vi "Basic Interface.vi"() -> ()   [LabVIEW 2019]
uses:
  source code/LSL components/scripts/scripts manager/scripts manager.lvclass
  source code/LSL components/output terminal/Plain OT/PainOutputTerminal.lvclass
  C:/Users/Patrick/Documents/GitHub/LabVIEW-Script-Language/source code/LSL components/output terminal/Base/Output Terminal.lvclass
  source code/LSL components/output terminal/Plain OT/PainOutputTerminal.lvclass/PainOutputTerminal.ctl
  source code/LSL components/variables/RT Variables/RT Variables.lvclass
  source code/LSL components/scripts/scripts manager/scripts manager.lvclass/scripts manager.ctl
  a3015e6c-1936-464d-a698-599e3c554b07.vi
  source code/LSL components/output terminal/Plain OT/properties/Write Output Terminal.vi
  source code/LSL components/scripts/scripts manager/properties/Write Scripts.vi
panel:
  in  "Script Editor":string
  in  "Path":path
  in  "Help":bool
  in  "Script Compile":bool
  in  "Script Save":bool
  in  "Script Delete":bool
  in  "Script New":bool
  in  "Script Run":bool
  in  "Script Files":i32(listbox)
  out "Output Terminal":string
  in  "Script Line":string
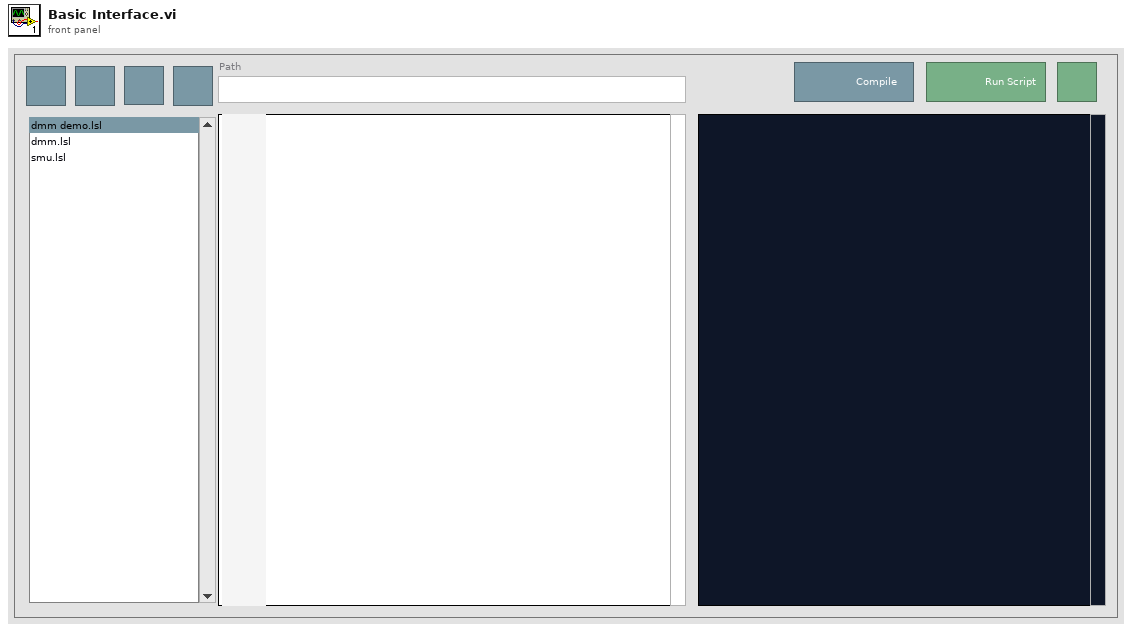
[diagram p1: front panel]
types:
  T1 = enum32{"Invalid", "Standard", "Closed", "Hidden", "Minimized", "Maximized"}
  T2 = enum32{"invalid app kind", "Development System", "Run Time System", "Student Edition", "Embedded LabVIEW", "Evaluation", "Custom"}
  T3 = cluster{"Core":cluster{"Current VI Reference":refnum<vi>, "Close Panel on Exit?":bool}, "scripts manager":refnum<class "scripts manager.lvclass">, "Script":string, "Script Folder":path, "Script Filename":string, "PainOT":refnum<class "PainOutputTerminal.lvclass">}
  T4 = cluster{"Current VI Reference":refnum<vi>, "Close Panel on Exit?":bool}
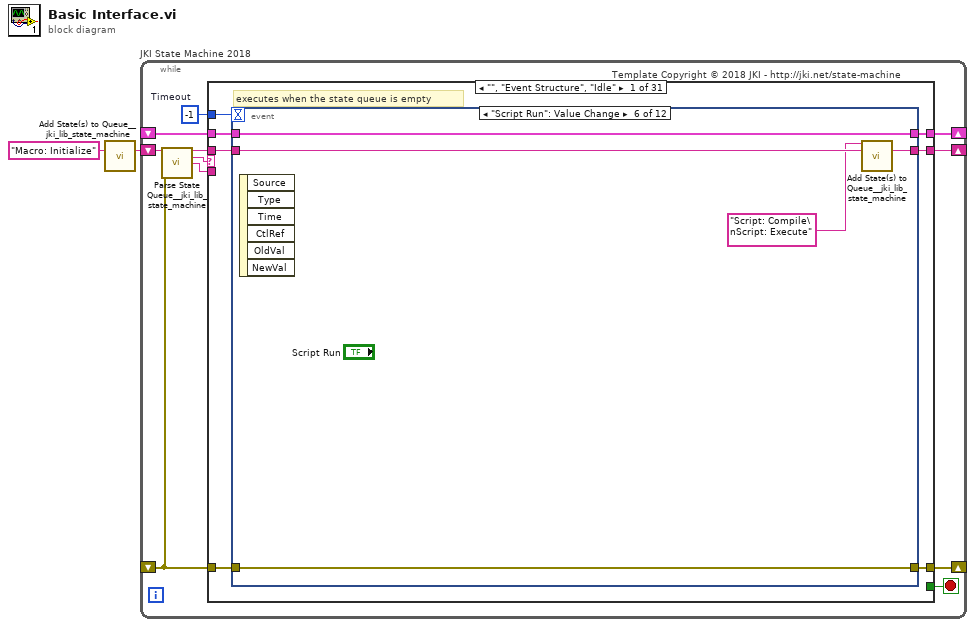
[diagram p0: block diagram]
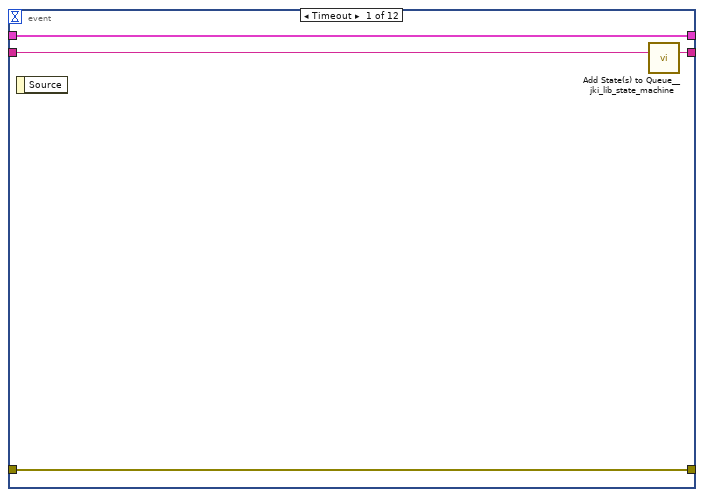
[diagram p2: hidden frame]
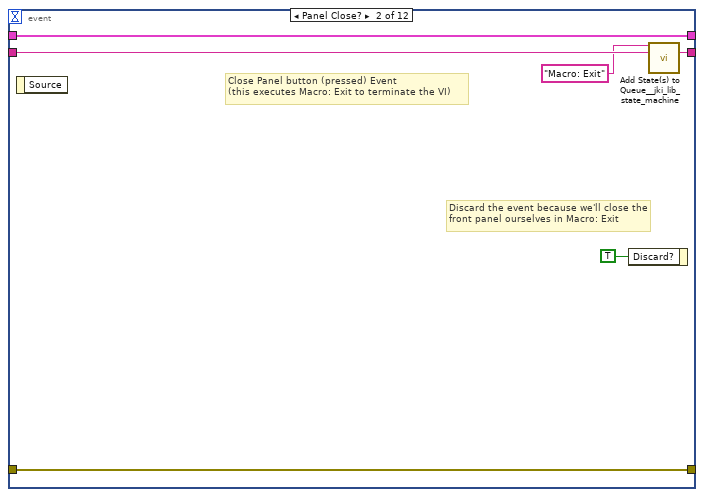
[diagram p3: hidden frame]
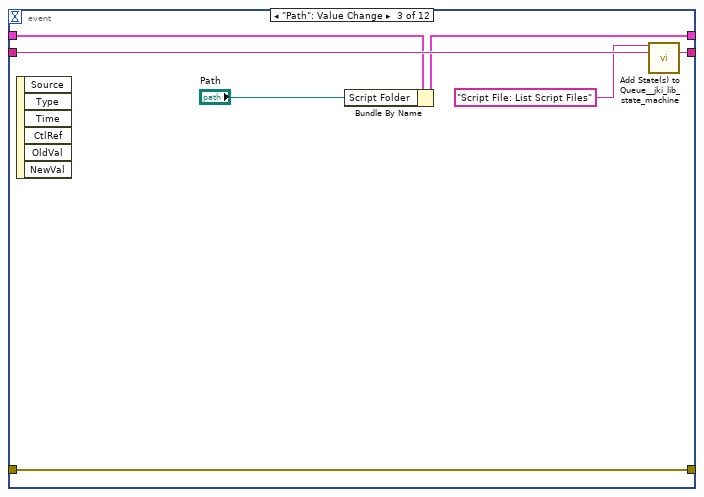
[diagram p4: hidden frame]
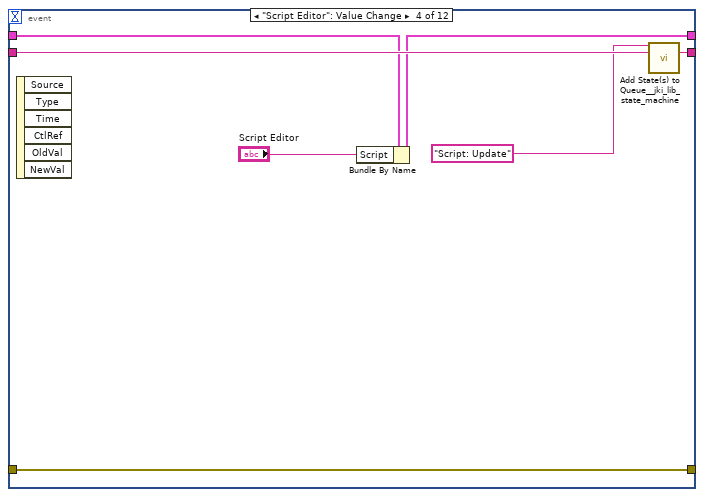
[diagram p5: hidden frame]
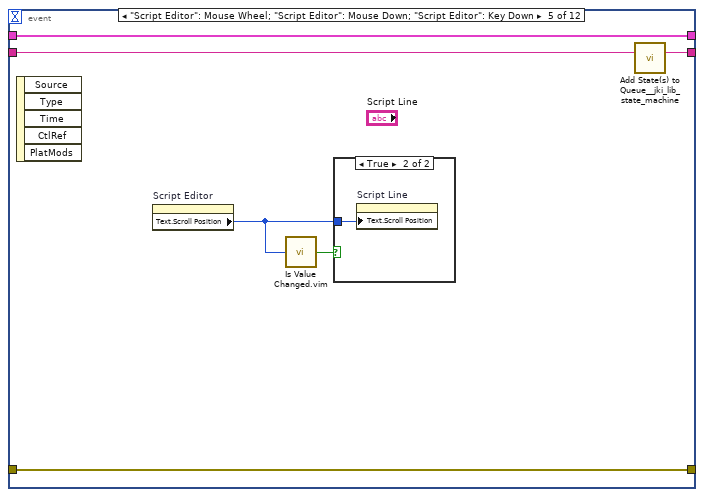
[diagram p6: hidden frame]
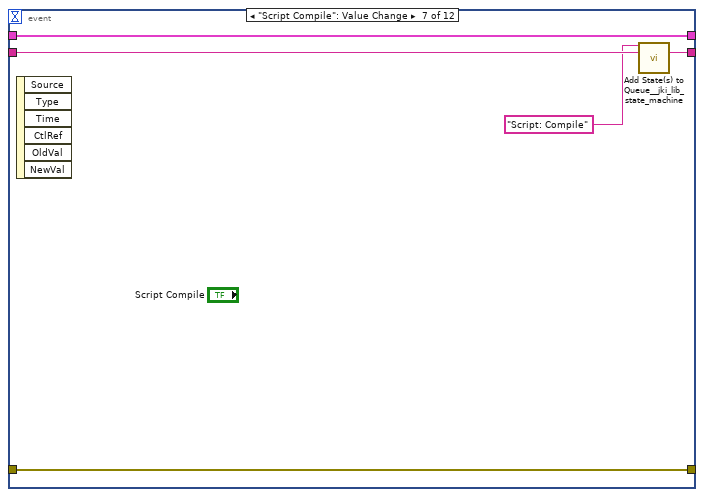
[diagram p8: hidden frame]
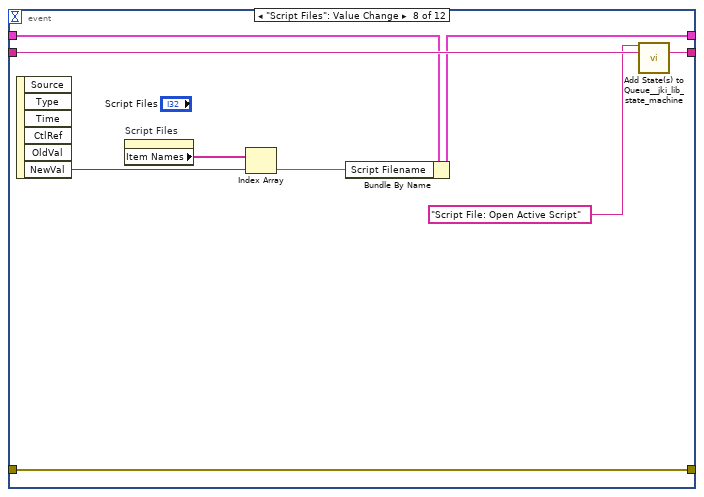
[diagram p9: hidden frame]
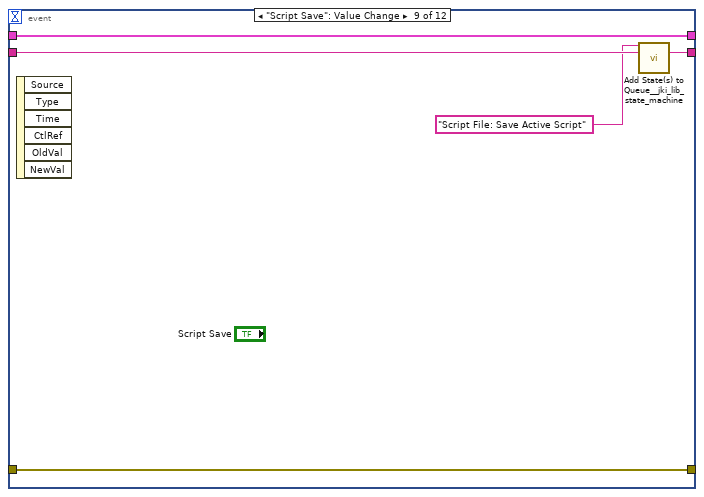
[diagram p10: hidden frame]
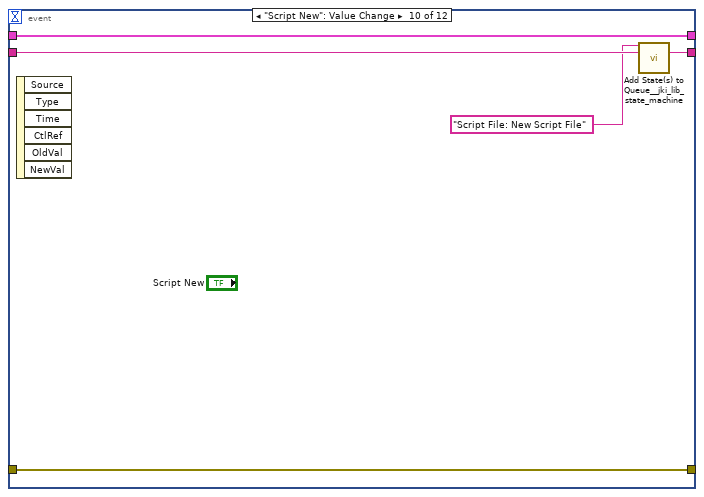
[diagram p11: hidden frame]
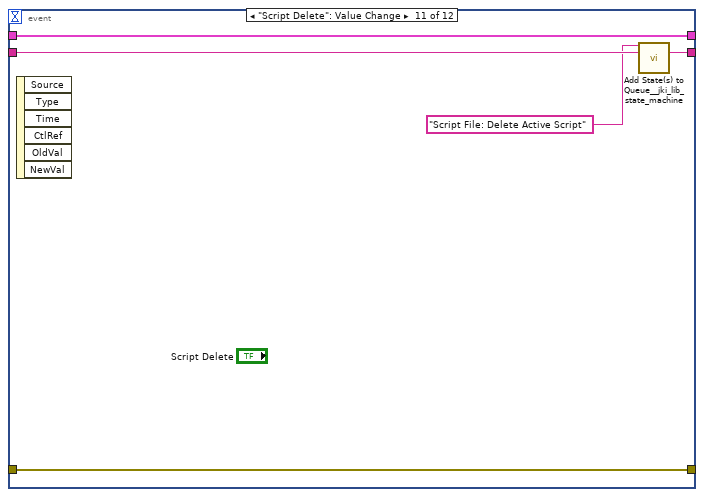
[diagram p12: hidden frame]
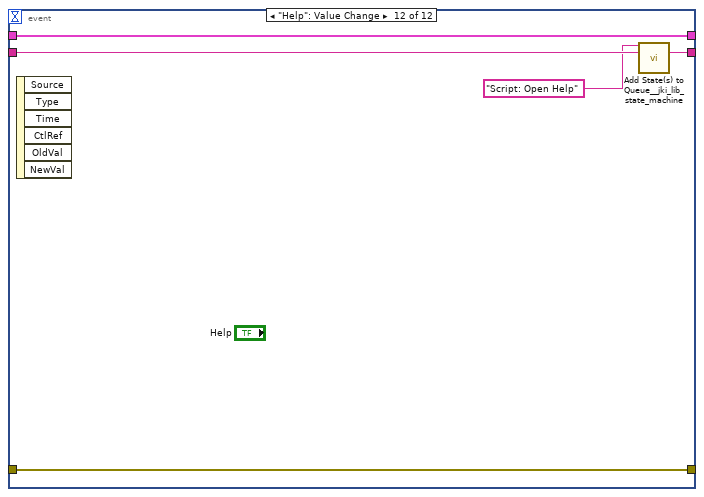
[diagram p13: hidden frame]
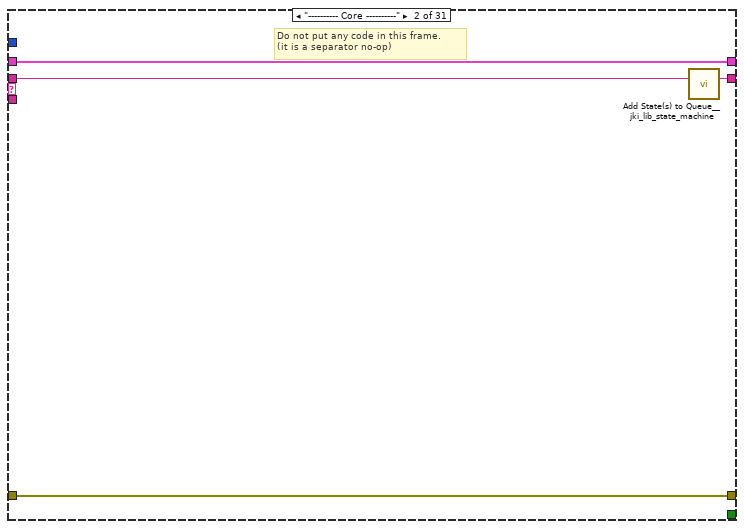
[diagram p14: hidden frame]
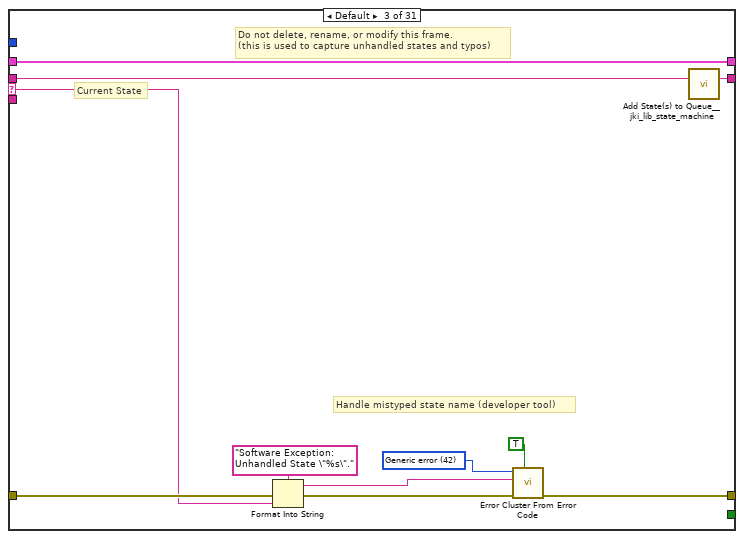
[diagram p15: hidden frame]
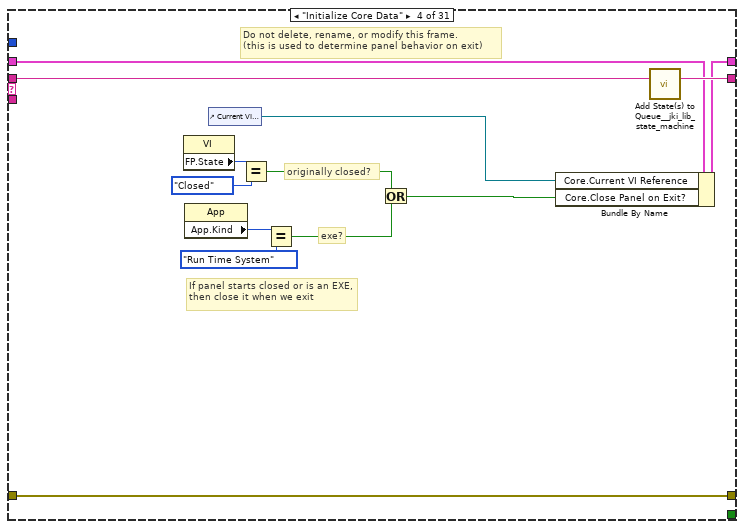
[diagram p16: hidden frame]
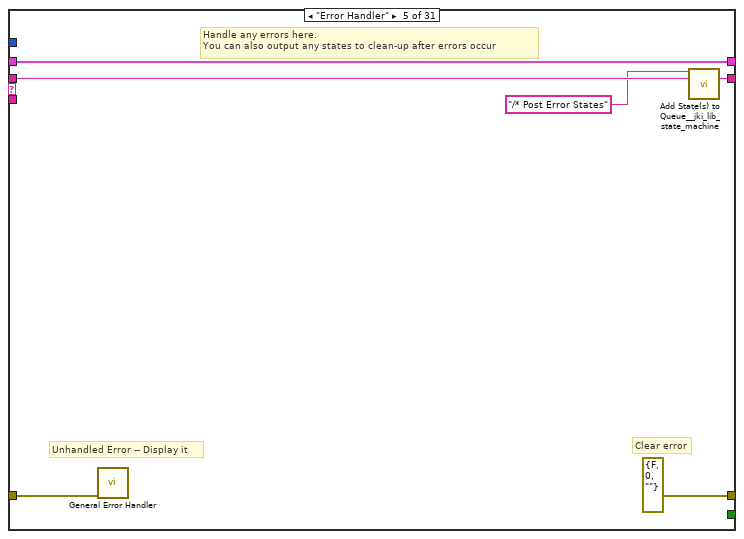
[diagram p17: hidden frame]
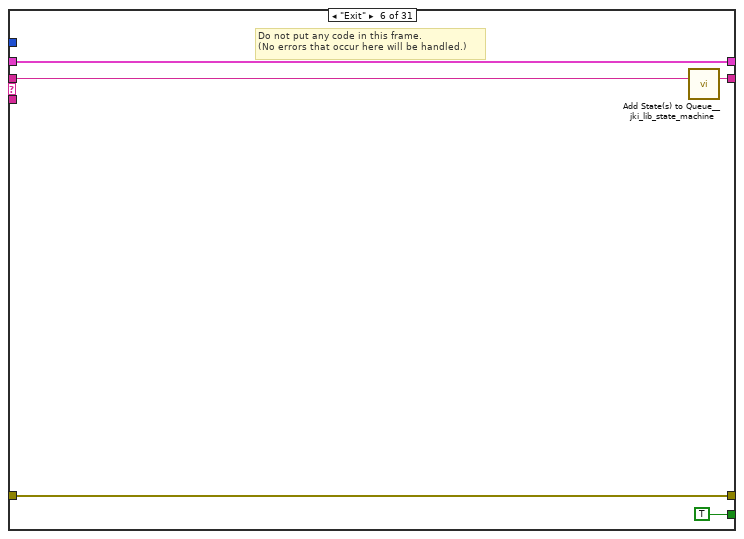
[diagram p18: hidden frame]
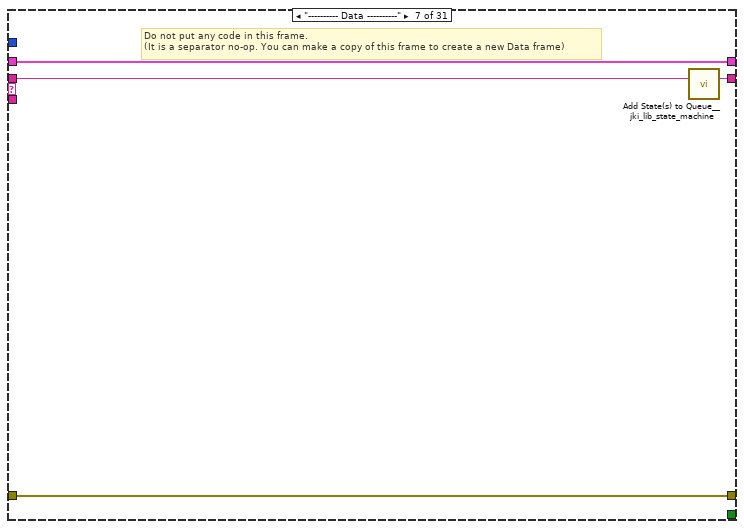
[diagram p19: hidden frame]
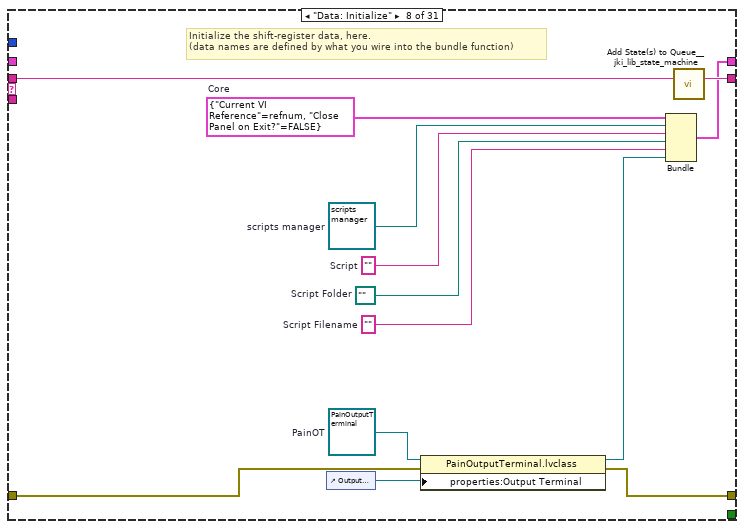
[diagram p20: hidden frame]
diagram:
  n1 = call <vilib>:"Add State(s) to Queue__jki_lib_state_machine.vi"("State(s) in (\"\")"="Macro: Initialize") -> ("States Out"=w2:string)  [unwired: 14 in]
  n2 = while "JKI State Machine 2018" {
    shift-right: [w6] -> _
    shift-left: _ -> [w5]
    shift-right: [w9] -> _
    shift-left: _ -> [w3]
    shift-right: [w8] -> _
    shift-left: w2 -> [w10]
    stop <- w7 stop-if-true
    w4 = -1  # Timeout
    # "Template Copyright © 2018 JKI - http://jki.net/state-machine"
    n3 = call <vilib>:"Parse State Queue__jki_lib_state_machine.vi"("State Queue"=w10, "Error In (no error)"=w3) -> ("Remaining States"=w12:string, "Current State"=w13:string, "Arguments"=w11:string)  [unwired: 11 in]
    n4 = case shown="\"\", \"Event Structure\", \"Idle\"" w13 {
      selector: w13 -> [_ _ w95 _ _ _ _ _ _ _ _ _ _ _ _ _ _ _ _ _ _ _ _ _ _ _ _ _ _ _ _]
      tunnel: w12 -> [w20 w94 w99 w118 w124 w129 w133 w146 w162 w187 w191 w203 w209 w220 w289 w294 w304 w310 w320 w329 w337 w345 w353 w358 w362 w373 w446 w456 w466 w478 w499]
      tunnel: w11 -> [_ _ _ _ _ _ _ _ _ _ _ _ w204 w214 _ _ _ _ _ _ _ _ _ _ _ w367 _ _ _ _ _]
      tunnel: w5 -> [w18 w91 w97 w111 w121 w127 w130 _ w151 w182 w188 w201 w207 w216 w286 w291 w301 w306 w317 w326 w334 w342 w350 w356 w359 w366 w444 w454 w464 w476 w497]
      tunnel: [w17 w92 w101 w115 errorcluster {"status"=FALSE, "code"=0, "source"=""} ("error out") w126 w131 w139 w150 w183 w189 w194 w205 w217 w287 w292 w302 w308 w314 w322 w332 w341 w347 w355 w360 w364 w438 w449 w462 w471 w491] -> w9
      tunnel: w3 -> [w16 w92 w100 w115 w120 w126 w131 w138 w149 w184 w189 w193 w206 w218 w287 w292 w302 w308 w313 w321 w331 w339 w346 w354 w360 w363 w437 w448 w457 w470 w490]
      tunnel: [w19 w93 w98 w117 w123 w128 w132 w145 w161 w186 w190 w202 w208 w219 w288 w293 w303 w309 w319 w328 w336 w344 w352 w357 w361 w372 w445 w455 w465 w477 w498] -> w8
      tunnel: [_ _ _ _ _ TRUE _ _ _ _ _ _ _ _ _ _ _ _ _ _ _ _ _ _ _ _ _ _ _ _ _] -> w7
      tunnel: [w15 w91 w97 w116 w121 w127 w130 w144 w152 w182 w188 w201 w207 w216 w286 w291 w301 w307 w318 w327 w335 w343 w351 w356 w359 w366 w444 w454 w464 w476 w497] -> w6
      tunnel: w4 -> [w14 _ _ _ _ _ _ _ _ _ _ _ _ _ _ _ _ _ _ _ _ _ _ _ _ _ _ _ _ _ _]
      frame "", "Event Structure", "Idle" {
        # "executes when the state queue is empty"
        n5 = event shown="[5] \"Script Run\": Value Change" {
          selector: _ -> [_ _ _ _ _ _ _ _ _ _ _ _]
          dyn-events: _ -> [_ _ _ _ _ _ _ _ _ _ _ _]
          timeout: w14 -> [_ _ _ _ _ _ _ _ _ _ _ _]
          tunnel: w20 -> [w24 w30 w37 w44 w49 w54 w59 w69 w73 w78 w83 w88]
          tunnel: [w23 w29 w36 w43 w50 w55 w60 w70 w74 w79 w84 w89] -> w19
          tunnel: w18 -> [w21 w27 w32 w39 w48 w56 w61 w65 w75 w80 w85 w90]
          tunnel: [w22 w28 w35 w42 w47 w52 w57 w67 w71 w76 w81 w86] -> w17
          tunnel: w16 -> [w22 w28 w35 w42 w47 w52 w57 w67 w71 w76 w81 w86]
          tunnel: [w21 w27 w33 w40 w48 w56 w61 w66 w75 w80 w85 w90] -> w15
          event Timeout {
            n6 = event-data() -> ()  [unwired: 1 in, 1 out]
            n7 = call <vilib>:"Add State(s) to Queue__jki_lib_state_machine.vi"("State(s) in (\"\")"=w24) -> ("States Out"=w23:string)  [unwired: 14 in]
          }
          event Panel Close? {
            # "Discard the event because we'll close the front panel ourselves in Macro: Exit"
            # "Close Panel button (pressed) Event\n(this executes Macro: Exit to terminate the VI)"
            n8 = event-data() -> ()  [unwired: 1 in, 1 out]
            n9 = event-data("Discard?"=TRUE) -> ()  [unwired: 1 in, 1 out]
            n10 = call <vilib>:"Add State(s) to Queue__jki_lib_state_machine.vi"("State(s) in Front (\"\")"="Macro: Exit", "State(s) in (\"\")"=w30) -> ("States Out"=w29:string)  [unwired: 13 in]
          }
          event "Path": Value Change {
            n11 = event-data() -> ()  [unwired: 1 in, 6 out]
            n12 = Bundle By Name(cluster=w32, "Script Folder"="Path") -> (w33:T3)
            n13 = call <vilib>:"Add State(s) to Queue__jki_lib_state_machine.vi"("State(s) in Front (\"\")"="Script File: List Script Files", "State(s) in (\"\")"=w37) -> ("States Out"=w36:string)  [unwired: 13 in]
          }
          event "Script Editor": Value Change {
            n14 = event-data() -> ()  [unwired: 1 in, 6 out]
            n15 = Bundle By Name(cluster=w39, "Script"="Script Editor") -> (w40:T3)
            n16 = call <vilib>:"Add State(s) to Queue__jki_lib_state_machine.vi"("State(s) in Front (\"\")"="Script: Update", "State(s) in (\"\")"=w44) -> ("States Out"=w43:string)  [unwired: 13 in]
          }
          event "Script Editor": Mouse Wheel; "Script Editor": Mouse Down; "Script Editor": Key Down {
            n17 = event-data() -> ()  [unwired: 1 in, 5 out]
            n18 = property on="Script Editor" class="Str"() -> ("Text.Scroll Position"=w46:u32)  [unwired: 2 in, 2 out]
            n19 = call "Is Value Changed.vim"("value"=w46) -> ("changed or first call?"=w45:bool)
            n20 = case shown="True" w45 {
              tunnel: w46 -> [_ w51]
              frame False {
              }
              frame True {
                n21 = property on="Script Line" class="Str"("Text.Scroll Position"=w51) -> ()  [unwired: 2 in, 2 out]
              }
            }
            n22 = call <vilib>:"Add State(s) to Queue__jki_lib_state_machine.vi"("State(s) in (\"\")"=w49) -> ("States Out"=w50:string)  [unwired: 14 in]
          }
          event "Script Run": Value Change {
            n23 = event-data() -> ()  [unwired: 1 in, 6 out]
            n24 = call <vilib>:"Add State(s) to Queue__jki_lib_state_machine.vi"("State(s) in Front (\"\")"="Script: Compile\nScript: Execute" ("State(s) at Back (\"\")"), "State(s) in (\"\")"=w54) -> ("States Out"=w55:string)  [unwired: 13 in]
          }
          event "Script Compile": Value Change {
            n25 = event-data() -> ()  [unwired: 1 in, 6 out]
            n26 = call <vilib>:"Add State(s) to Queue__jki_lib_state_machine.vi"("State(s) in Front (\"\")"="Script: Compile" ("State(s) at Back (\"\")"), "State(s) in (\"\")"=w59) -> ("States Out"=w60:string)  [unwired: 13 in]
          }
          event "Script Files": Value Change {
            n27 = event-data() -> ("NewVal"=w62:i32)  [unwired: 1 in, 5 out]
            n28 = property on="Script Files" class="LstBox (strict)"() -> ("Item Names"=w64:string[])  [unwired: 2 in, 2 out]
            n29 = Index Array(array=w64, index=w62) -> (element=w63:string)
            n30 = Bundle By Name(cluster=w65, "Script Filename"=w63) -> (w66:T3)
            n31 = call <vilib>:"Add State(s) to Queue__jki_lib_state_machine.vi"("State(s) in Front (\"\")"="Script File: Open Active Script" ("State(s) at Back (\"\")"), "State(s) in (\"\")"=w69) -> ("States Out"=w70:string)  [unwired: 13 in]
          }
          event "Script Save": Value Change {
            n32 = event-data() -> ()  [unwired: 1 in, 6 out]
            n33 = call <vilib>:"Add State(s) to Queue__jki_lib_state_machine.vi"("State(s) in Front (\"\")"="Script File: Save Active Script" ("State(s) at Back (\"\")"), "State(s) in (\"\")"=w73) -> ("States Out"=w74:string)  [unwired: 13 in]
          }
          event "Script New": Value Change {
            n34 = event-data() -> ()  [unwired: 1 in, 6 out]
            n35 = call <vilib>:"Add State(s) to Queue__jki_lib_state_machine.vi"("State(s) in Front (\"\")"="Script File: New Script File" ("State(s) at Back (\"\")"), "State(s) in (\"\")"=w78) -> ("States Out"=w79:string)  [unwired: 13 in]
          }
          event "Script Delete": Value Change {
            n36 = event-data() -> ()  [unwired: 1 in, 6 out]
            n37 = call <vilib>:"Add State(s) to Queue__jki_lib_state_machine.vi"("State(s) in Front (\"\")"="Script File: Delete Active Script" ("State(s) at Back (\"\")"), "State(s) in (\"\")"=w83) -> ("States Out"=w84:string)  [unwired: 13 in]
          }
          event "Help": Value Change {
            n38 = event-data() -> ()  [unwired: 1 in, 6 out]
            n39 = call <vilib>:"Add State(s) to Queue__jki_lib_state_machine.vi"("State(s) in Front (\"\")"="Script: Open Help" ("State(s) at Back (\"\")"), "State(s) in (\"\")"=w88) -> ("States Out"=w89:string)  [unwired: 13 in]
          }
        }
      }
      frame "---------- Core ----------" {
        # "Do not put any code in this frame.\n(it is a separator no-op)"
        n40 = call <vilib>:"Add State(s) to Queue__jki_lib_state_machine.vi"("State(s) in (\"\")"=w94) -> ("States Out"=w93:string)  [unwired: 14 in]
      }
      frame Default {
        w104 = 42 items=["No error", "Argument error", "Memory is full", "Out of zone", "End of file", "File already open", "Generic file I/O error", "File not found", "File permission error", "Disk is full", "Duplicate path", "Too many files open", "System feature not enabled", "Resource file not found", "Cannot add resource", "Resource not found", "Image not found", "Image memory error", "Pen does not exist", "Config type invalid", "Config token not found", "Config parse error", "Config memory error", "Bad external code format", "Bad external code offset", "External code not present", "Null window", "Destroy window error", "Null menu", "Print aborted", "Bad print record", "Print driver error", "Windows error during printing", "Memory error during printing", "Print dialog error", "Generic print error", "Invalid device refnum", "Device not found", "Device parameter error", "Device unit error", "Cannot open device", "Device call aborted", "Generic error", "Cancelled by user", "Object ID too low", "Object ID too high", "Object not in heap", "Unknown heap", "Unknown object (invalid DefProc)", "Unknown object (DefProc not in table)", "Message out of range", "Invalid (null) method", "Unknown message", "Manager call not supported", "Bad address", "Network operation in progress", "Network operation timed out", "Connection is busy", "Network attribute not supported", "Network error", "Address in use", "System out of memory", "Connection aborted", "Connection refused", "Not connected", "Already connected", "Connection closed", "Initialization error (interapplication manager)", "Bad occurrence", "Wait on unbound occurrence handler", "Occurrence queue overflow", "Datalog type conflict", "Unused", "Unrecognized type (interapplication manager)", "Memory corrupt", "Failed to make temporary DLL", "Old CIN version", "Drag socket not found", "Failed to load drop-object", "Failed to register OLE object", "Failed to release OLE object", "Format specifier type mismatch", "Unknown format specifier", "Too few format specifiers", "Too many format specifiers", "Scan failed", "Newer CIN version", "Error converting to variant", "Runtime menu error", "Password tampered", "Variant attribute not found", "Incompatible variant data type", "Event data is not available", "Event Store is not present", "Occurrence is not found", "Event Queue is not created", "Event info is not available", "Refnum passed is NULL", "Error retrieving Class GUID", "Error retrieving CoClass GUID", "Error retrieving TypeLib GUID.", "Bad built application magic bytes.", "Specific driver is different from the specific driver associated with the Logical Name.", "There is no session opened to the class driver.", "Max Error", "MAX - Error with config objects", "MAX - Error loading configuration", "MAX - Group not supported"]
        # "Current State"
        # "Do not delete, rename, or modify this frame.\n(this is used to capture unhandled states and typos)"
        # "Handle mistyped state name (developer tool)"
        n41 = Format Into String(format string="Software Exception: Unhandled State \"%s\"." ("message"), error in=w100, w95) -> (resulting string=w103:string, error out=w102:errorcluster)  [unwired: 1 in]
        n42 = call <vilib>:"Error Cluster From Error Code.vi"("show call chain? (False)"=TRUE, "error in (no error)"=w102, "error message (\"\")"=w103, "error code (0)"=w104) -> ("error out"=w101:errorcluster)  [unwired: 5 in]
        n43 = call <vilib>:"Add State(s) to Queue__jki_lib_state_machine.vi"("State(s) in (\"\")"=w99) -> ("States Out"=w98:string)  [unwired: 14 in]
      }
      frame "Initialize Core Data" {
        # "Do not delete, rename, or modify this frame.\n(this is used to determine panel behavior on exit)"
        # "originally closed?"
        # "exe?"
        # "If panel starts closed or is an EXE, then close it when we exit"
        n44 = property class="VI"() -> ("FP.State"=w108:T1)  [unwired: 2 in, 2 out]
        n45 = property class="App"() -> ("App.Kind"=w114:T2)  [unwired: 2 in, 2 out]
        n46 = control-ref of="Current VI Reference"() -> (w109:refnum<vi>)
        n47 = Equal?(x=w108, y=T1."Closed" ("Front Panel Window:State")) -> (x = y?=w106:bool)
        n48 = Equal?(x=w114, y=T2."Run Time System" ("Application:Kind")) -> (x = y?=w112:bool)
        n49 = Or(x=w106, y=w112) -> (x .or. y?=w110:bool)
        n50 = Bundle By Name(cluster=w111, "Core.Current VI Reference"=w109, "Core.Close Panel on Exit?"=w110) -> (w116:T3)
        n51 = call <vilib>:"Add State(s) to Queue__jki_lib_state_machine.vi"("State(s) in (\"\")"=w118) -> ("States Out"=w117:string)  [unwired: 14 in]
      }
      frame "Error Handler" {
        # "Unhandled Error -- Display it"
        # "Handle any errors here.\nYou can also output any states to clean-up after errors occur"
        # "Clear error"
        n52 = call <vilib>:"General Error Handler.vi"("error in (no error)"=w120) -> ()  [unwired: 10 in, 5 out]
        n53 = call <vilib>:"Add State(s) to Queue__jki_lib_state_machine.vi"("State(s) in Front (\"\")"="/* Post Error States", "State(s) in (\"\")"=w124) -> ("States Out"=w123:string)  [unwired: 13 in]
      }
      frame "Exit" {
        # "Do not put any code in this frame.\n(No errors that occur here will be handled.)"
        n54 = call <vilib>:"Add State(s) to Queue__jki_lib_state_machine.vi"("State(s) in (\"\")"=w129) -> ("States Out"=w128:string)  [unwired: 14 in]
      }
      frame "---------- Data ----------" {
        # "Do not put any code in this frame.\n(It is a separator no-op. You can make a copy of this frame to create a new Data frame)"
        n55 = call <vilib>:"Add State(s) to Queue__jki_lib_state_machine.vi"("State(s) in (\"\")"=w133) -> ("States Out"=w132:string)  [unwired: 14 in]
      }
      frame "Data: Initialize" {
        w134 = ""  # Script Filename
        w135 = path ""  # Script Folder
        w141 = refnum<class "PainOutputTerminal.lvclass"> refnum  # PainOT
        w136 = ""  # Script
        w137 = refnum<class "scripts manager.lvclass"> refnum  # scripts manager
        w143 = T4 {"Current VI Reference"=refnum, "Close Panel on Exit?"=FALSE}  # Core
        # "Initialize the shift-register data, here.\n(data names are defined by what you wire into the bundle function)"
        n56 = control-ref of="Output Terminal"() -> (w142:refnum<vi>)
        n57 = property class="PainOutputTerminal.lvclass"(reference=w141, error in=w138, "properties:Output Terminal"=w142) -> (reference out=w140:refnum<class "PainOutputTerminal.lvclass">, error out=w139:errorcluster)
        n58 = Bundle("Core"=w143, "scripts manager"=w137, "Script"=w136, "Script Folder"=w135, "Script Filename"=w134, "PainOT"=w140) -> (w144:T3)  [unwired: 1 in]
        n59 = call <vilib>:"Add State(s) to Queue__jki_lib_state_machine.vi"("State(s) in (\"\")"=w146) -> ("States Out"=w145:string)  [unwired: 14 in]
      }
      frame "Data: Configure defaults" {
        # "Do not put any code in this frame.\n(It is a separator no-op. You can make a copy of this frame to create a new Data frame)"
        n60 = disable-structure shown="Default" {
          disable-tunnel: [w163 w167] -> w160
          frame condition #0 (active) {
            n61 = Current VI's Path() -> (path=w166:path)
            n62 = Strip Path(path=w166) -> (stripped path=w165:path)  [unwired: 1 out]
            n63 = Build Path(base path=w165, name or relative path="lsl files") -> (appended path=w163:path)
          }
          frame condition #1 {
            n64 = call <vilib>:"Application Directory.vi"() -> ("Application Directory"=w168:path)
            n65 = Build Path(base path=w168, name or relative path="script files") -> (appended path=w167:path)
          }
        }
        n66 = for {
          N: 100 -> [_]
          tunnel: [w174] -> w157 mode=indexing
          i -> [w175]
          n67 = Increment(x=w175) -> (x+1=w174:i32)
        }
        n68 = Number To Decimal String(number=w157) -> (decimal integer string=w159:string[])  [unwired: 1 in]
        n69 = for {
          tunnel: w159 -> [w170] mode=indexing
          shift-right: [w173] -> w158
          shift-left: "" -> [w171]
          n70 = Concatenate Strings(w171, w170, "\n") -> (w173:string)
        }
        n71 = call <vilib>:"Check if File or Folder Exists.vi"("error in (no error)"=w149, "path"=w160) -> ("error out"=w155:errorcluster, "file or folder exists?"=w153:bool, "dup path"=w154:path)  [unwired: 7 in]
        n72 = case shown="False" w153 {
          tunnel: w155 -> [w179 w180]
          tunnel: w154 -> [w178 w181]
          tunnel: [w176 w181] -> w148
          tunnel: [w177 w180] -> w150
          frame False {
            n73 = Create Folder(path (use dialog)=w178, error in=w179) -> (created path=w176:path, error out=w177:errorcluster)  [unwired: 1 in, 1 out]
          }
          frame True {
          }
        }
        n74 = property on="Script Line" class="Str"("Value"=w158) -> ()  [unwired: 2 in, 2 out]
        n75 = local write "Path"(w148) -> ()
        n76 = Bundle By Name(cluster=w151, "Script Folder"=w148) -> (w152:T3)
        n77 = call <vilib>:"Add State(s) to Queue__jki_lib_state_machine.vi"("State(s) in (\"\")"=w162) -> ("States Out"=w161:string)  [unwired: 14 in]
      }
      frame "Data: Cleanup" {
        # "Cleanup any data and references, here.\n(this is called automatically, by the Macro: Exit)"
        n78 = Unbundle By Name(w182) -> ("Core.Current VI Reference"=w185:refnum<vi>)
        n79 = Close Reference(reference=w185, error in (no error)=w184) -> (error out=w183:errorcluster)
        n80 = call <vilib>:"Add State(s) to Queue__jki_lib_state_machine.vi"("State(s) in (\"\")"=w187) -> ("States Out"=w186:string)  [unwired: 14 in]
      }
      frame "---------- UI ----------" {
        # "Do not put any code in this frame.\n(It is a separator no-op. You can make a copy of this frame to create a new UI frame)"
        n81 = call <vilib>:"Add State(s) to Queue__jki_lib_state_machine.vi"("State(s) in (\"\")"=w191) -> ("States Out"=w190:string)  [unwired: 14 in]
      }
      frame "UI: Initialize" {
        w192 = "" ("Output Terminal")
        w197 = u32 923176
        # "Initialize the User Interface, here.\n(this is called automatically, by the Macro: Init)"
        n82 = local write "Output Terminal"(w192) -> ()
        n83 = local write "Script Editor"(w192) -> ()
        n84 = local write "Script Line"(w192) -> ()
        n85 = property on="Script Files" class="LstBox (strict)"("Item Names"=string[] []) -> ()  [unwired: 2 in, 2 out]
        n86 = property on="Output Terminal" class="Str"("Text.BG Color"=w197, "Text.BGColor"=w197, "Text.TextColor"=u32 16777215) -> ()  [unwired: 2 in, 2 out]
        n87 = property on="Script Line" class="Str"("Text.BG Color"=u32 16119285) -> ()  [unwired: 2 in, 2 out]
        n88 = property on="Script Files" class="LstBox (strict)"("SelColor"=u32 8034469) -> ()  [unwired: 2 in, 2 out]
        n89 = call <userlib>:"Fit VI window to Largest Dec__ogtk.vi"("error in (no error)"=w193, "border spacing (2 px)"=0) -> ("error out"=w194:errorcluster)  [unwired: 4 in, 1 out]
        n90 = call <vilib>:"Add State(s) to Queue__jki_lib_state_machine.vi"("State(s) in (\"\")"=w203) -> ("States Out"=w202:string)  [unwired: 14 in]
        "Output Terminal" <- w192
      }
      frame "UI: Cursor Set" {
        # "Argument"
        # "Set and Unset Cursor Busy.\n(Usage: \"UI: Cursor Set >> Busy|Idle\")"
        n91 = case shown="\"Idle\", Default" w204 {
          tunnel: w206 -> [w211 w213]
          tunnel: [w210 w212] -> w205
          frame "Idle", Default {
            n92 = call <vilib>:"Unset Busy.vi"("error in (no error)"=w211) -> ("error out"=w210:errorcluster)  [unwired: 10 in]
          }
          frame "Busy" {
            n93 = call <vilib>:"Set Busy.vi"("error in (no error)"=w213) -> ("error out"=w212:errorcluster)  [unwired: 9 in, 1 out]
          }
        }
        n94 = call <vilib>:"Add State(s) to Queue__jki_lib_state_machine.vi"("State(s) in (\"\")"=w209) -> ("States Out"=w208:string)  [unwired: 14 in]
      }
      frame "UI: Front Panel State" {
        # "Argument"
        # "Set Front Panel Open or Closed\n(Usage: \"UI: Front Panel State >> Open|Close\")"
        n95 = Unbundle By Name(w216) -> ("Core.Current VI Reference"=w215:refnum<vi>)
        n96 = case shown="\"Minimize\", \"Minimized\"" w214 {
          tunnel: w218 -> [w226 w241 w252 w265 w278]
          tunnel: [w228 w242 w254 w267 w280] -> w217
          tunnel: w215 -> [w227 w239 w253 w266 w279]
          frame "Open", "Standard", Default {
            w221 = T1."Standard" ("State")
            n97 = property class="VI"(reference=w227, error in=w226) -> (reference out=w224:refnum<vi>, error out=w225:errorcluster, "FP.State"=w223:T1)
            n98 = Not Equal?(x=w223, y=w221) -> (x != y?=w222:bool)
            n99 = case shown="True" w222 {
              tunnel: [w232 w234] -> w228
              tunnel: w225 -> [w231 w234]
              tunnel: w224 -> [w230 _]
              tunnel: w221 -> [w229 _]
              frame True {
                n100 = invoke class="VI" method="FP.Open"(reference=w230, error in=w231, "Activate"=TRUE, "State"=w229) -> (error out=w232:errorcluster)  [unwired: 1 in, 4 out]
              }
              frame False {
              }
            }
          }
          frame "Close", "Closed" {
            n101 = property class="VI"(reference=w239, error in=w241) -> (reference out=w238:refnum<vi>, error out=w240:errorcluster, "FP.State"=w236:T1)
            n102 = Not Equal?(x=w236, y=T1."Closed" ("Front Panel Window:State")) -> (x != y?=w235:bool)
            n103 = case shown="True" w235 {
              tunnel: [w243 w246] -> w242
              tunnel: w240 -> [w243 w245]
              tunnel: w238 -> [_ w244]
              frame False {
              }
              frame True {
                n104 = invoke class="VI" method="FP.Close"(reference=w244, error in=w245) -> (error out=w246:errorcluster)  [unwired: 1 in, 2 out]
              }
            }
          }
          frame "Hidden", "Hide" {
            w247 = T1."Hidden" ("State")
            n105 = property class="VI"(reference=w253, error in=w252) -> (reference out=w250:refnum<vi>, error out=w251:errorcluster, "FP.State"=w249:T1)
            n106 = Not Equal?(x=w249, y=w247) -> (x != y?=w248:bool)
            n107 = case shown="True" w248 {
              tunnel: [w258 w259] -> w254
              tunnel: w251 -> [w257 w259]
              tunnel: w250 -> [w256 _]
              tunnel: w247 -> [w255 _]
              frame True {
                n108 = invoke class="VI" method="FP.Open"(reference=w256, error in=w257, "State"=w255) -> (error out=w258:errorcluster)  [unwired: 2 in, 4 out]
              }
              frame False {
              }
            }
          }
          frame "Minimize", "Minimized" {
            w260 = T1."Minimized" ("State")
            n109 = property class="VI"(reference=w266, error in=w265) -> (reference out=w263:refnum<vi>, error out=w264:errorcluster, "FP.State"=w262:T1)
            n110 = Not Equal?(x=w262, y=w260) -> (x != y?=w261:bool)
            n111 = case shown="True" w261 {
              tunnel: [w271 w272] -> w267
              tunnel: w264 -> [w270 w272]
              tunnel: w263 -> [w269 _]
              tunnel: w260 -> [w268 _]
              frame True {
                n112 = invoke class="VI" method="FP.Open"(reference=w269, error in=w270, "State"=w268) -> (error out=w271:errorcluster)  [unwired: 2 in, 4 out]
              }
              frame False {
              }
            }
          }
          frame "Maximize", "Maximized" {
            w273 = T1."Maximized" ("State")
            n113 = property class="VI"(reference=w279, error in=w278) -> (reference out=w276:refnum<vi>, error out=w277:errorcluster, "FP.State"=w275:T1)
            n114 = Not Equal?(x=w275, y=w273) -> (x != y?=w274:bool)
            n115 = case shown="True" w274 {
              tunnel: [w284 w285] -> w280
              tunnel: w277 -> [w283 w285]
              tunnel: w276 -> [w282 _]
              tunnel: w273 -> [w281 _]
              frame True {
                n116 = invoke class="VI" method="FP.Open"(reference=w282, error in=w283, "State"=w281) -> (error out=w284:errorcluster)  [unwired: 2 in, 4 out]
              }
              frame False {
              }
            }
          }
        }
        n117 = call <vilib>:"Add State(s) to Queue__jki_lib_state_machine.vi"("State(s) in (\"\")"=w220) -> ("States Out"=w219:string)  [unwired: 14 in]
      }
      frame "---------- Macro ----------" {
        # "Do not put any code in this frame.\n(It is a separator no-op. You can make a copy of this frame to create a new Macro frame)"
        n118 = call <vilib>:"Add State(s) to Queue__jki_lib_state_machine.vi"("State(s) in (\"\")"=w289) -> ("States Out"=w288:string)  [unwired: 14 in]
      }
      frame "Macro: Initialize" {
        w290 = "Data: Initialize\nInitialize Core Data\nUI: Initialize\nUI: Front Panel State >> Open\n\nData: Configure defaults\n\nScript: Init\nScript File: List Script Files\nScript File: Open Active Script"  # Data: Initialize Initialize Core Data UI: Initialize UI: Front Panel State >> Open  Data: Configure defaults  Script: Init Script File: List Script Files Script File: Open Active Script
        # "Initialization Macro\n(This is called once, when the VI starts)"
        n119 = call <vilib>:"Add State(s) to Queue__jki_lib_state_machine.vi"("State(s) in Front (\"\")"=w290, "State(s) in (\"\")"=w294) -> ("States Out"=w293:string)  [unwired: 13 in]
      }
      frame "Macro: Exit" {
        # "Exit Macro\n(This is called once, when the VI exits)"
        n120 = Unbundle By Name(w301) -> ("Core.Close Panel on Exit?"=w300:bool)
        n121 = Select(t="UI: Front Panel State >> Close", s=w300, f="") -> (s? t:f=w297:string)
        n122 = call <vilib>:"Add State(s) to Queue__jki_lib_state_machine.vi"("State(s) in (\"\")"=w297, "State(s) at Back (\"\")"="Data: Cleanup\n\nScript: Close\n\nExit") -> ("States Out"=w295:string)  [unwired: 13 in]
        n123 = call <vilib>:"Add State(s) to Queue__jki_lib_state_machine.vi"("State(s) in Front (\"\")"=w295, "State(s) in (\"\")"=w304) -> ("States Out"=w303:string)  [unwired: 13 in]
      }
      frame "---------- Script ----------" {
        # "Script Template Separator\n(You can make a copy of, or modify, this frame)"
        n124 = Unbundle By Name(w306) -> ("scripts manager"=w305:refnum<class "scripts manager.lvclass">)  [unwired: 2 out]
        n125 = Bundle By Name(cluster=w306, "scripts manager"=w305) -> (w307:T3)
        n126 = call <vilib>:"Add State(s) to Queue__jki_lib_state_machine.vi"("State(s) in (\"\")"=w310) -> ("States Out"=w309:string)  [unwired: 14 in]
      }
      frame "Script: Init" {
        w315 = refnum<class "RT Variables.lvclass"> refnum  # RT Variables
        w316 = refnum<class "scripts manager.lvclass"> refnum  # scripts manager
        # "Script Template Separator\n(You can make a copy of, or modify, this frame)"
        n127 = Unbundle By Name(w317) -> ("PainOT"=w311:refnum<class "PainOutputTerminal.lvclass">)  [unwired: 2 out]
        n128 = call-dynamic "Instantiate.vi"("scripts manager in"=w316, "Output Terminal"=w311, "RT Variables"=w315, "error in (no error)"=w313) -> ("scripts manager out"=w312:refnum<class "scripts manager.lvclass">, "error out"=w314:errorcluster)  [unwired: 10 in]
        n129 = Bundle By Name(cluster=w317, "scripts manager"=w312) -> (w318:T3)
        n130 = call <vilib>:"Add State(s) to Queue__jki_lib_state_machine.vi"("State(s) in (\"\")"=w320) -> ("States Out"=w319:string)  [unwired: 14 in]
      }
      frame "Script: Update" {
        # "Script Template Separator\n(You can make a copy of, or modify, this frame)"
        n131 = Unbundle By Name(w326) -> ("Script"=w325:string, "scripts manager"=w324:refnum<class "scripts manager.lvclass">)  [unwired: 1 out]
        n132 = property class="scripts manager.lvclass"(reference=w324, error in=w321, "properties:Scripts"=w325) -> (reference out=w323:refnum<class "scripts manager.lvclass">, error out=w322:errorcluster)
        n133 = Bundle By Name(cluster=w326, "scripts manager"=w323) -> (w327:T3)
        n134 = call <vilib>:"Add State(s) to Queue__jki_lib_state_machine.vi"("State(s) in (\"\")"=w329) -> ("States Out"=w328:string)  [unwired: 14 in]
      }
      frame "Script: Compile" {
        # "Script Template Separator\n(You can make a copy of, or modify, this frame)"
        n135 = Unbundle By Name(w334) -> ("scripts manager"=w333:refnum<class "scripts manager.lvclass">)  [unwired: 2 out]
        n136 = call-dynamic "Compile Script.vi"("scripts manager in"=w333, "error in (no error)"=w331) -> ("scripts manager out"=w330:refnum<class "scripts manager.lvclass">, "error out"=w332:errorcluster)  [unwired: 12 in]
        n137 = Bundle By Name(cluster=w334, "scripts manager"=w330) -> (w335:T3)
        n138 = call <vilib>:"Add State(s) to Queue__jki_lib_state_machine.vi"("State(s) in (\"\")"=w337) -> ("States Out"=w336:string)  [unwired: 14 in]
      }
      frame "Script: Execute" {
        # "Script Template Separator\n(You can make a copy of, or modify, this frame)"
        n139 = Unbundle By Name(w342) -> ("scripts manager"=w340:refnum<class "scripts manager.lvclass">)  [unwired: 2 out]
        n140 = call-dynamic "Execute Script.vi"("scripts manager in"=w340, "error in (no error)"=w339) -> ("scripts manager out"=w338:refnum<class "scripts manager.lvclass">, "error out"=w341:errorcluster)  [unwired: 12 in]
        n141 = Bundle By Name(cluster=w342, "scripts manager"=w338) -> (w343:T3)
        n142 = call <vilib>:"Add State(s) to Queue__jki_lib_state_machine.vi"("State(s) in (\"\")"=w345) -> ("States Out"=w344:string)  [unwired: 14 in]
      }
      frame "Script: Close" {
        # "Script Template Separator\n(You can make a copy of, or modify, this frame)"
        n143 = Unbundle By Name(w350) -> ("scripts manager"=w349:refnum<class "scripts manager.lvclass">)  [unwired: 2 out]
        n144 = call-dynamic "Destroy.vi"("scripts manager in"=w349, "error in (no error)"=w346) -> ("scripts manager out"=w348:refnum<class "scripts manager.lvclass">, "error out"=w347:errorcluster)  [unwired: 12 in]
        n145 = Bundle By Name(cluster=w350, "scripts manager"=w348) -> (w351:T3)
        n146 = call <vilib>:"Add State(s) to Queue__jki_lib_state_machine.vi"("State(s) in (\"\")"=w353) -> ("States Out"=w352:string)  [unwired: 14 in]
      }
      frame "Script: Open Help" {
        # "Template Separator\n(You can make a copy of, or modify, this frame)"
        n147 = call "Open CHM documentation.vi"("error in"=w354) -> ("error out"=w355:errorcluster)  [unwired: 10 in]
        n148 = call <vilib>:"Add State(s) to Queue__jki_lib_state_machine.vi"("State(s) in (\"\")"=w358) -> ("States Out"=w357:string)  [unwired: 14 in]
      }
      frame "---------- Script File ----------" {
        # "Script File Template Separator\n(You can make a copy of, or modify, this frame)"
        n149 = Unbundle By Name(w359) -> ()  [unwired: 2 out]
        n150 = call <vilib>:"Add State(s) to Queue__jki_lib_state_machine.vi"("State(s) in (\"\")"=w362) -> ("States Out"=w361:string)  [unwired: 14 in]
      }
      frame "Script: File Operations" {
        # "Your code here.\n(You can make a copy of, or modify, this frame)"
        n151 = property on="Script Files" class="LstBox (strict)"() -> ("Item Names"=w370:string[], "Value"=w371:i32)  [unwired: 2 in, 2 out]
        n152 = Unbundle By Name(w366) -> ("Script Folder"=w369:path, "Script"=w368:string)
        n153 = Index Array(array=w370, index=w371) -> (element=w365:string)
        n154 = case shown="\"New Script File\"" w367 {
          tunnel: w363 -> [w374 w384 w390 w397 w403 w426]
          tunnel: [w374 w381 w388 w395 w407 w421] -> w364
          tunnel: w368 -> [_ _ _ w394 _ _]
          tunnel: w365 -> [_ _ w386 w393 w405 _]
          tunnel: w369 -> [_ w375 w385 w392 w406 _]
          tunnel: w370 -> [_ _ _ _ w401 w422]
          tunnel: [_ _ _ _ w399 w418] -> _
          tunnel: w371 -> [_ _ _ _ w400 _]
          frame Default {
          }
          frame "List Script File" {
            n155 = List Folder(path=w375, pattern="*.lsl", error in=w384) -> (filenames=w378:string[], error out=w382:errorcluster)  [unwired: 1 in, 2 out]
            n156 = Empty Array?(array=w378) -> (empty?=w379:bool)
            n157 = Select(t=string[] ["main.lsl"], s=w379, f=w378) -> (s? t:f=w377:string[])
            n158 = property on="Script Files" class="LstBox (strict)"(error in=w382, "Item Names"=w377, "Value"=0 ("Files")) -> (error out=w381:errorcluster)  [unwired: 1 in, 1 out]
          }
          frame "Open Active Script" {
            n159 = Build Path(base path=w385, name or relative path=w386) -> (appended path=w391:path)
            n160 = Read from Text File(file (use dialog)=w391, error in=w390) -> (text=w387:string, error out=w389:errorcluster)  [unwired: 2 in, 2 out]
            n161 = property on="Script Editor" class="Str"("Val(Sgnl)"=w387) -> ()  [unwired: 2 in, 2 out]
            n162 = call <vilib>:"Clear Errors.vi"("error in (no error)"=w389) -> ("error out"=w388:errorcluster)  [unwired: 5 in, 1 out]
          }
          frame "Save Active Script" {
            n163 = Build Path(base path=w392, name or relative path=w393) -> (appended path=w398:path)
            n164 = Write to Text File(file (use dialog)=w398, text=w394, error in=w397) -> (error out=w396:errorcluster)  [unwired: 1 in, 2 out]
            n165 = call <vilib>:"Clear Errors.vi"("error in (no error)"=w396) -> ("error out"=w395:errorcluster)  [unwired: 5 in, 1 out]
          }
          frame "Delete Active Script" {
            n166 = Build Path(base path=w406, name or relative path=w405) -> (appended path=w404:path)
            n167 = case shown="Default" w405 {
              tunnel: w404 -> [w415 _]
              tunnel: w403 -> [w416 w417]
              tunnel: [w414 w417] -> w402
              tunnel: w401 -> [w413 _]
              tunnel: w400 -> [w410 _]
              tunnel: ["Script: File Operations >> Open Active Script" _] -> w399
              frame Default {
                n168 = Delete From Array(array=w413, length=1, index=w410) -> (array with subset deleted=w412:string[])  [unwired: 1 out]
                n169 = Delete(path (use dialog)=w415, error in=w416) -> (error out=w414:errorcluster)  [unwired: 3 in, 2 out]
                n170 = property on="Script Files" class="LstBox (strict)"("Item Names"=w412, "Value"=0 ("Script Files")) -> ()  [unwired: 2 in, 2 out]
              }
              frame "main.lsl" {
              }
            }
            n171 = call <vilib>:"Clear Errors.vi"("error in (no error)"=w402) -> ("error out"=w407:errorcluster)  [unwired: 5 in, 1 out]
          }
          frame "New Script File" {
            n172 = call "New Script File2"("error in (no error)"=w426) -> ("File Name"=w423:string, "Create"=w424:bool, "error out"=w425:errorcluster)  [unwired: 16 in]
            n173 = Concatenate Strings(w423, ".lsl" ("string")) -> (w420:string)
            n174 = case shown="True" w424 {
              tunnel: w425 -> [w427 w429]
              tunnel: w420 -> [_ w433]
              tunnel: w422 -> [_ w431]
              tunnel: [w427 w429] -> w421
              tunnel: [_ "Script: File Operations >> Open Active Script"] -> w418
              frame False {
              }
              frame True {
                n175 = Build Array (concatenate)(w431, w433) -> (w432:string[])
                n176 = Array Size(array=w431) -> (size(s)=w430:i32)
                n177 = property on="Script Files" class="LstBox (strict)"("Item Names"=w432, "Value"=w430) -> ()  [unwired: 2 in, 2 out]
              }
            }
          }
        }
        n178 = call <vilib>:"Add State(s) to Queue__jki_lib_state_machine.vi"("State(s) in (\"\")"=w373) -> ("States Out"=w372:string)  [unwired: 14 in]
      }
      frame "Script File: List Script Files" {
        # "Script File Template Separator\n(You can make a copy of, or modify, this frame)"
        n179 = Unbundle By Name(w444) -> ("Script Folder"=w439:path)  [unwired: 1 out]
        n180 = List Folder(path=w439, pattern="*.lsl", error in=w437) -> (filenames=w435:string[], error out=w443:errorcluster)  [unwired: 1 in, 2 out]
        n181 = Empty Array?(array=w435) -> (empty?=w442:bool)
        n182 = Select(t=string[] ["main.lsl"], s=w442, f=w435) -> (s? t:f=w441:string[])
        n183 = property on="Script Files" class="LstBox (strict)"(error in=w443, "Item Names"=w441, "Value"=0 ("Files")) -> (error out=w438:errorcluster)  [unwired: 1 in, 1 out]
        n184 = call <vilib>:"Add State(s) to Queue__jki_lib_state_machine.vi"("State(s) in (\"\")"=w446) -> ("States Out"=w445:string)  [unwired: 14 in]
      }
      frame "Script File: Open Active Script" {
        # "Script File Template Separator\n(You can make a copy of, or modify, this frame)"
        n185 = Unbundle By Name(w454) -> ("Script Folder"=w451:path, "Script Filename"=w450:string)
        n186 = Build Path(base path=w451, name or relative path=w450) -> (appended path=w453:path)
        n187 = Read from Text File(file (use dialog)=w453, error in=w448) -> (text=w452:string, error out=w447:errorcluster)  [unwired: 2 in, 2 out]
        n188 = call <vilib>:"Clear Errors.vi"("error in (no error)"=w447) -> ("error out"=w449:errorcluster)  [unwired: 5 in, 1 out]
        n189 = property on="Script Editor" class="Str"("Val(Sgnl)"=w452) -> ()  [unwired: 2 in, 2 out]
        n190 = call <vilib>:"Add State(s) to Queue__jki_lib_state_machine.vi"("State(s) in (\"\")"=w456) -> ("States Out"=w455:string)  [unwired: 14 in]
      }
      frame "Script File: Save Active Script" {
        # "Script File Template Separator\n(You can make a copy of, or modify, this frame)"
        n191 = Unbundle By Name(w464) -> ("Script Folder"=w460:path, "Script Filename"=w461:string, "Script"=w459:string)
        n192 = Build Path(base path=w460, name or relative path=w461) -> (appended path=w463:path)
        n193 = Write to Text File(file (use dialog)=w463, text=w459, error in=w457) -> (error out=w458:errorcluster)  [unwired: 1 in, 2 out]
        n194 = call <vilib>:"Clear Errors.vi"("error in (no error)"=w458) -> ("error out"=w462:errorcluster)  [unwired: 5 in, 1 out]
        n195 = call <vilib>:"Add State(s) to Queue__jki_lib_state_machine.vi"("State(s) in (\"\")"=w466) -> ("States Out"=w465:string)  [unwired: 14 in]
      }
      frame "Script File: Delete Active Script" {
        # "Script File Template Separator\n(You can make a copy of, or modify, this frame)"
        n196 = Unbundle By Name(w476) -> ("Script Folder"=w473:path, "Script Filename"=w472:string)
        n197 = property on="Script Files" class="LstBox (strict)"() -> ("Item Names"=w469:string[], "Value"=w468:i32)  [unwired: 2 in, 2 out]
        n198 = Index Array(array=w469, index=w468) -> (element=w467:string)
        n199 = Build Path(base path=w473, name or relative path=w472) -> (appended path=w475:path)
        n200 = case shown="Default" w467 {
          tunnel: w475 -> [w486 _]
          tunnel: w470 -> [w487 w488]
          tunnel: [w485 w488] -> w474
          tunnel: w469 -> [w484 _]
          tunnel: w468 -> [w481 _]
          tunnel: ["Script File: Open Active Script" _] -> _
          frame Default {
            n201 = Delete From Array(array=w484, length=1, index=w481) -> (array with subset deleted=w483:string[])  [unwired: 1 out]
            n202 = Delete(path (use dialog)=w486, error in=w487) -> (error out=w485:errorcluster)  [unwired: 3 in, 2 out]
            n203 = property on="Script Files" class="LstBox (strict)"("Item Names"=w483, "Value"=0 ("Script Files")) -> ()  [unwired: 2 in, 2 out]
          }
          frame "main.lsl" {
          }
        }
        n204 = call <vilib>:"Clear Errors.vi"("error in (no error)"=w474) -> ("error out"=w471:errorcluster)  [unwired: 5 in, 1 out]
        n205 = call <vilib>:"Add State(s) to Queue__jki_lib_state_machine.vi"("State(s) in (\"\")"=w478) -> ("States Out"=w477:string)  [unwired: 14 in]
      }
      frame "Script File: New Script File" {
        # "Script File Template Separator\n(You can make a copy of, or modify, this frame)"
        n206 = property on="Script Files" class="LstBox (strict)" props=["Item Names", "Value"]() -> ("Item Names"=w489:string[])  [unwired: 2 in, 3 out]
        n207 = Unbundle By Name(w497) -> ()  [unwired: 2 out]
        n208 = call "New Script File"("error in (no error)"=w490) -> ("File Name"=w494:string, "Create"=w495:bool, "error out"=w496:errorcluster)  [unwired: 16 in]
        n209 = Concatenate Strings(w494, ".lsl" ("string")) -> (w493:string)
        n210 = case shown="True" w495 {
          tunnel: w496 -> [w500 w502]
          tunnel: w493 -> [_ w506]
          tunnel: w489 -> [_ w504]
          tunnel: [w500 w502] -> w491
          tunnel: [_ "Script File: Open Active Script"] -> _
          frame False {
          }
          frame True {
            n211 = Build Array (concatenate)(w504, w506) -> (w505:string[])
            n212 = Array Size(array=w504) -> (size(s)=w503:i32)
            n213 = property on="Script Files" class="LstBox (strict)"("Item Names"=w505, "Value"=w503) -> ()  [unwired: 2 in, 2 out]
          }
        }
        n214 = call <vilib>:"Add State(s) to Queue__jki_lib_state_machine.vi"("State(s) in (\"\")"=w499) -> ("States Out"=w498:string)  [unwired: 14 in]
      }
    }
  }
